vi "run_diff.vi"(11 "Command Line":string[](array[string])) -> (2 "stdout | stderr":string, 3 "Return Code":i32)   [LabVIEW 2020]
uses:
  <vilib>/Utility/error.llb/DialogType.ctl
  <vilib>/Utility/error.llb/Error Cluster From Error Code.vi
  <vilib>/ErrorRing/Error Ring.xnode
  DiffVI/Modules/Screenshots/VIDiffScreenshots.lvlib
panel:
  out "Full Report":string
  out "All Diffs Succeeded":bool
  out "error out":errorcluster
  # "Required by LabVIEWCLI\n(via connector pane)"
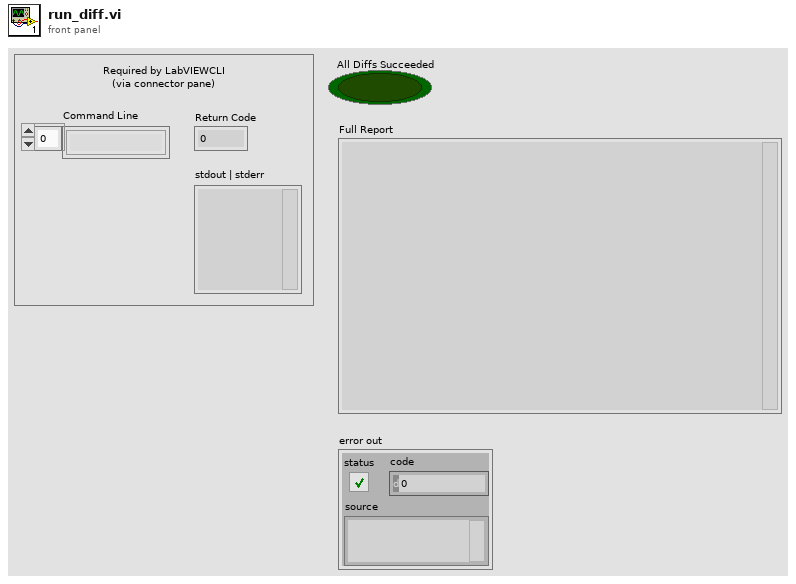
[diagram p1: front panel]
types:
  T1 = typedef "DialogType.ctl" = u16
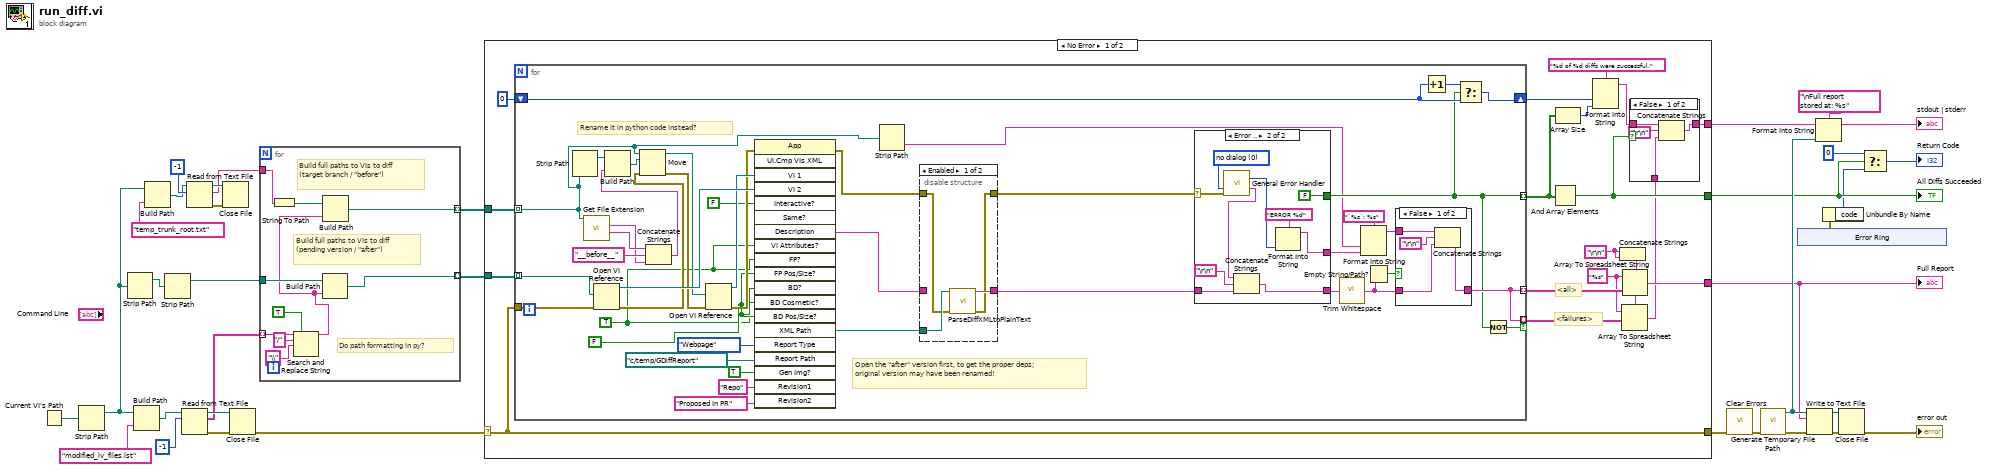
[diagram p0: block diagram]
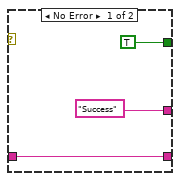
[diagram p5: hidden frame]
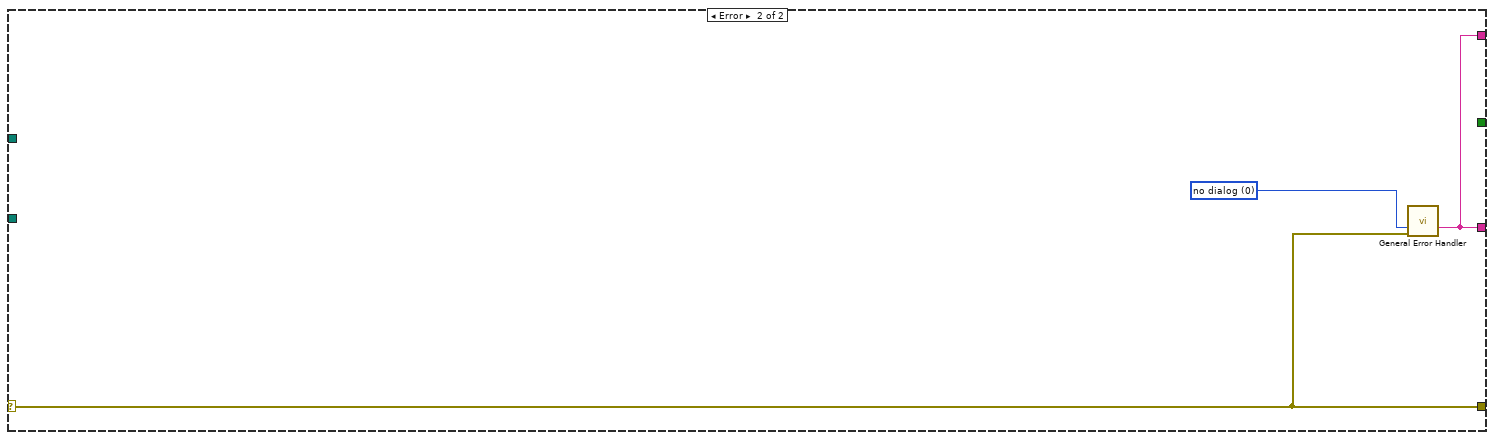
[diagram p6: hidden frame]
diagram:
  n1 = Current VI's Path() -> (path=w35:path)
  n2 = Strip Path(path=w35) -> (stripped path=w8:path)  [unwired: 1 out]
  n3 = Strip Path(path=w8) -> (stripped path=w13:path)  [unwired: 1 out]
  n4 = Build Path(base path=w8, name or relative path="modified_lv_files.lst") -> (appended path=w15:path)
  n5 = Build Path(base path=w8, name or relative path="temp_trunk_root.txt") -> (appended path=w5:path)
  n6 = Strip Path(path=w13) -> (stripped path=w11:path)  [unwired: 1 out]
  n7 = Read from Text File(file (use dialog)=w15, count=-1) -> (refnum out=w17:refnum<file>, text=w14:string[], error out=w18:errorcluster)  [unwired: 2 in, 1 out]
  n8 = Read from Text File(file (use dialog)=w5, count=-1) -> (refnum out=w3:refnum<file>, text=w2:string, error out=w4:errorcluster)  [unwired: 2 in, 1 out]
  n9 = Close File(refnum=w3, error in=w4) -> ()  [unwired: 2 out]
  n10 = Close File(refnum=w17, error in=w18) -> (error out=w12:errorcluster)  [unwired: 1 out]
  n11 = for {
    tunnel: w11 -> [w44]
    tunnel: w14 -> [w39] mode=indexing
    tunnel: [w45] -> w10 mode=indexing
    tunnel: w2 -> [w43]
    tunnel: [w41] -> w1 mode=indexing
    # "Do path formatting in py?"
    # "Build full paths to VIs to diff (target branch / \"before\")"
    # "Build full paths to VIs to diff (pending version / \"after\")"
    n12 = String To Path(string=w43) -> (path=w42:path)
    n13 = Search and Replace String(replace all?=TRUE ("replace all? (F)"), input string=w39, search string="/", replace string="\\" ("replace string (\"\")")) -> (result string=w40:string)  [unwired: 4 in, 3 out]
    n14 = Build Path(base path=w44, name or relative path=w40) -> (appended path=w45:path)
    n15 = Build Path(base path=w42, name or relative path=w40) -> (appended path=w41:path)
  }
  n16 = case shown="No Error" w12 {
    selector: w12 -> [w62 w136]
    tunnel: w10 -> [w63 _]
    tunnel: [w62 w136] -> w34
    tunnel: [w55 _] -> w25
    tunnel: [w52 w134] -> w26
    tunnel: [w53 w134] -> w31
    tunnel: w1 -> [w46 _]
    frame No Error {
      w48 = "%s" ("format string")
      w61 = "\r\n"
      # "<failures>"
      # "<all>"
      n17 = for {
        tunnel: w63 -> [w102] mode=indexing
        tunnel: w62 -> [w109]
        tunnel: [w104] -> w57 mode=indexing
        tunnel: [w108] -> w51 mode=indexing
        tunnel: [w108] -> w50 mode=indexing if=w107
        shift-right: [w103] -> w58
        shift-left: 0 -> [w105]
        tunnel: w46 -> [w101] mode=indexing
        w75 = FALSE
        w74 = TRUE
        # "Rename it in python code instead?"
        # "Open the \"after\" version first, to get the proper deps; original version may have been renamed!"
        n18 = Strip Path(path=w101) -> (stripped path=w94:path)  [unwired: 1 out]
        n19 = call <vilib>:"Get File Extension.vi"("file"=w101) -> ("filename without extension"=w91:string, "lowercase file extension"=w90:string)  [unwired: 6 in, 3 out]
        n20 = Open VI Reference(vi path=w102, error in (no error)=w109) -> (vi reference=w100:refnum<vi>, error out=w80:errorcluster)  [unwired: 4 in]
        n21 = Concatenate Strings(w91, "__before__" ("string"), w90) -> (w89:string)
        n22 = Build Path(base path=w94, name or relative path=w89) -> (appended path=w88:path)
        n23 = Move(source path=w101, error in=w80, 10:w88) -> (error out=w79:errorcluster, 3:w92:path)  [unwired: 2 in, 1 out]
        n24 = Open VI Reference(vi path=w92, error in (no error)=w79) -> (vi reference=w99:refnum<vi>, error out=w95:errorcluster)  [unwired: 4 in]
        n25 = invoke class="App" method="UI.Cmp VIs XML"(error in=w95, "VI 1"=w99, "VI 2"=w100, "Interactive?"=FALSE, "VI Attributes?"=w74, "FP?"=w74, "FP Pos/Size?"=w75, "BD?"=w74, "BD Cosmetic?"=w75, "BD Pos/Size?"=w75, "Report Type"=enum32{"None", "Webpage", "Text", "MS Word"}."Webpage", "Report Path"=path "c:/temp/GDiffReport", "Gen Img?"=TRUE, "Revision1"="Repo", "Revision2"="Proposed In PR") -> (error out=w70:errorcluster, "Description"=w71:string, "XML Path"=w73:path)  [unwired: 5 in, 17 out]
        n26 = Strip Path(path=w101) -> (name=w81:string)  [unwired: 1 out]
        n27 = disable-structure shown="Enabled" {
          disable-tunnel: w73 -> [w113 _]
          disable-tunnel: [w112 w115] -> w72
          disable-tunnel: w71 -> [_ w115]
          disable-tunnel: w70 -> [w111 w114]
          disable-tunnel: [w110 w114] -> w69
          frame Enabled {
            n28 = call "ParseDiffXMLtoPlainText.vi"("XML Path"=w113, "error in"=w111) -> ("change description"=w112:string, "error out"=w110:errorcluster)  [unwired: 12 in]
          }
          frame Disabled {
          }
        }
        n29 = case shown="Error .." w69 {
          selector: w69 -> [_ w131]
          tunnel: ["Success" ("Control Name") w128] -> w86
          tunnel: [TRUE FALSE] -> w104
          tunnel: w72 -> [w123 w127]
          tunnel: [w123 w126] -> w85
          frame No Error {
          }
          frame Error {
            w132 = T1 0 items=["no dialog", "OK message", "continue or stop message", "OK message + warnings", "continue/stop + warnings"] ("type of dialog (OK msg:1)")
            n30 = call <vilib>:"General Error Handler.vi"("type of dialog (OK msg:1)"=w132, "error in (no error)"=w131) -> ("code out"=w130:i32, "message"=w125:string)  [unwired: 9 in, 3 out]
            n31 = Concatenate Strings(w125, "\r\n", w127) -> (w126:string)
            n32 = Format Into String(format string="ERROR %d", w130) -> (resulting string=w128:string)  [unwired: 2 in, 1 out]
          }
        }
        n33 = call <vilib>:"Trim Whitespace.vi"("string"=w85) -> ("trimmed string"=w84:string)  [unwired: 1 in]
        n34 = Format Into String(format string="`%s`: %s" ("Control Name"), w81, w86) -> (resulting string=w82:string)  [unwired: 2 in, 1 out]
        n35 = Empty String/Path?(string/path=w84) -> (empty?=w83:bool)
        n36 = case shown="False" w83 {
          tunnel: w84 -> [w118 _]
          tunnel: w82 -> [w119 w120]
          tunnel: [w117 w120] -> w108
          frame False {
            n37 = Concatenate Strings(w119, "\r\n", w118) -> (w117:string)
          }
          frame True {
          }
        }
        n38 = Increment(x=w105) -> (x+1=w106:i32)
        n39 = Select(t=w106, s=w104, f=w105) -> (s? t:f=w103:i32)
        n40 = Not(x=w104) -> (.not. x?=w107:bool)
      }
      n41 = And Array Elements(Boolean array=w57) -> (logical AND=w55:bool)
      n42 = Array Size(array=w57) -> (size(s)=w56:i32)
      n43 = Format Into String(format string="%d of %d diffs were successful." ("Control Name"), w58, w56) -> (resulting string=w54:string)  [unwired: 2 in, 1 out]
      n44 = Concatenate Strings(w61, w61) -> (w49:string)
      n45 = Array To Spreadsheet String(delimiter (Tab)=w49, array=w50, 3:w48) -> (spreadsheet string=w47:string)
      n46 = Array To Spreadsheet String(delimiter (Tab)=w49, array=w51, 3:w48) -> (spreadsheet string=w52:string)
      n47 = case shown="False" w55 {
        tunnel: w54 -> [w67 w68]
        tunnel: [w64 w68] -> w53
        tunnel: w47 -> [w65 _]
        frame False {
          n48 = Concatenate Strings(w67, "\r\n", w65) -> (w64:string)
        }
        frame True {
        }
      }
    }
    frame Error {
      w135 = T1 0 items=["no dialog", "OK message", "continue or stop message", "OK message + warnings", "continue/stop + warnings"] ("type of dialog (OK msg:1)")
      n49 = call <vilib>:"General Error Handler.vi"("type of dialog (OK msg:1)"=w135, "error in (no error)"=w136) -> ("message"=w134:string)  [unwired: 9 in, 4 out]
    }
  }
  "All Diffs Succeeded" <- w25
  "Full Report" <- w26
  n50 = call <vilib>:"Clear Errors.vi"("error in (no error)"=w34) -> ("error out"=w33:errorcluster)  [unwired: 5 in, 1 out]
  n51 = call <vilib>:"Generate Temporary File Path.vi"("error in (no error)"=w33) -> ("error out"=w28:errorcluster, "Unique Temporary File Path"=w29:path)  [unwired: 9 in]
  n52 = xnode "Error Ring"() -> ("error out"=w20:errorcluster)
  n53 = Write to Text File(file (use dialog)=w29, text=w26, error in=w28) -> (refnum out=w30:refnum<file>, error out=w27:errorcluster)  [unwired: 1 in, 1 out]
  n54 = Format Into String(format string="\nFull report stored at: %s" ("Control Name"), initial string=w31, w29) -> (resulting string=→"stdout | stderr":string)  [unwired: 1 in, 1 out]
  n55 = Unbundle By Name(w20) -> ("code"=w19:i32)
  n56 = Close File(refnum=w30, error in=w27) -> (error out=→"error out":errorcluster)  [unwired: 1 out]
  n57 = Select(t=0, s=w25, f=w19) -> (s? t:f=→"Return Code":i32)
